vi "action controller.vi"(10 "Box Sensor":bool, 11 "Buttons":bool[](array[boolean])) -> ()   [LabVIEW 2018]
uses:
  First Power Up 2018 current/Robot Global Data.vi
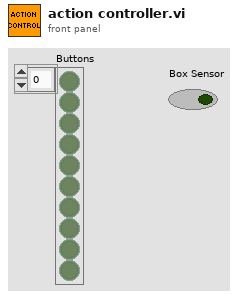
[diagram p1: front panel]
types:
  T1 = enum16{"Pickup", "Store", "Lift", "Straight Lift"}
  T2 = cluster{"Buttons[0]":bool, "Buttons[1]":bool, "Buttons[2]":bool, "Buttons[3]":bool, "Buttons[4]":bool, "Buttons[5]":bool, "Buttons[6]":bool, "Buttons[7]":bool, "Buttons[8]":bool}
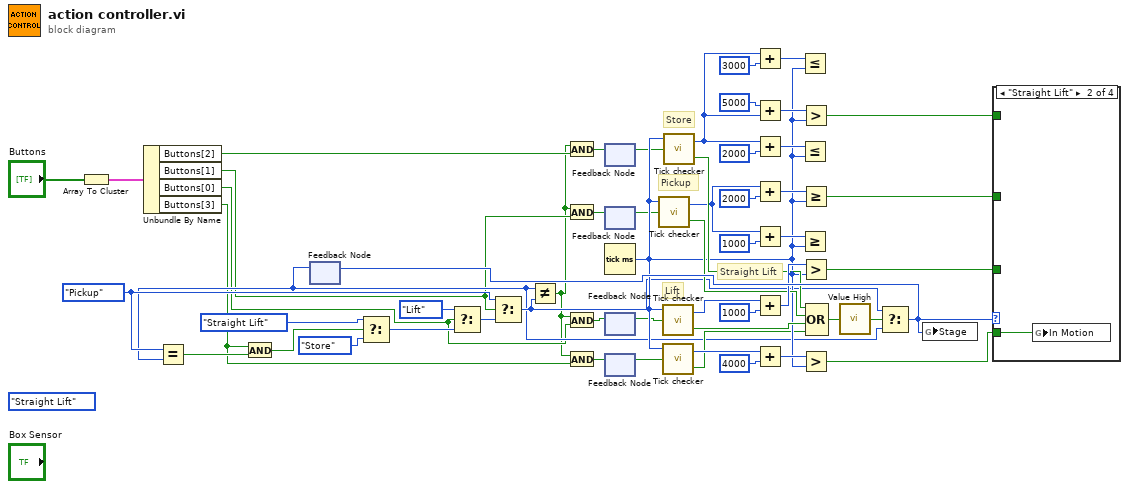
[diagram p0: block diagram]
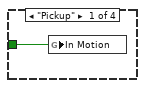
[diagram p2: hidden frame]
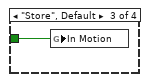
[diagram p3: hidden frame]
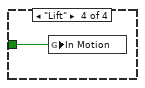
[diagram p4: hidden frame]
diagram:
  w44 = T1."Pickup" ("Stage")
  (unwired) T1."Straight Lift" ("Stage")
  # "Straight Lift"
  # "Lift"
  # "Pickup"
  # "Store"
  n1 = Array To Cluster(array="Buttons") -> (cluster=w54:T2)
  n2 = Unbundle By Name(w54) -> ("Buttons[2]"=w13:bool, "Buttons[1]"=w9:bool, "Buttons[0]"=w6:bool, "Buttons[3]"=w3:bool)
  n3 = feedback #1() -> (w14:T1)  [unwired: 1 in]
  n4 = Equal?(x=w44, y=w14) -> (x = y?=w46:bool)
  n5 = And(x=w3, y=w46) -> (x .and. y?=w45:bool)
  n6 = Select(t=T1."Straight Lift" ("Stage"), s=w45, f=T1."Store" ("Stage")) -> (s? t:f=w51:T1)
  n7 = Select(t=T1."Lift" ("Stage"), s=w6, f=w51) -> (s? t:f=w50:T1)
  n8 = Select(t=w44, s=w9, f=w50) -> (s? t:f=w15:T1)
  n9 = Not Equal?(x=w14, y=w15) -> (x != y?=w2:bool)
  n10 = And(x=w2, y=w13) -> (x .and. y?=w12:bool)
  n11 = And(x=w2, y=w9) -> (x .and. y?=w10:bool)
  n12 = And(x=w2, y=w6) -> (x .and. y?=w7:bool)
  n13 = And(x=w2, y=w3) -> (x .and. y?=w4:bool)
  n14 = feedback-in #2(w12) -> ()
  n15 = feedback #2() -> (w11:bool)  [unwired: 1 in]
  n16 = feedback #3() -> (w8:bool)  [unwired: 1 in]
  n17 = feedback-in #3(w10) -> ()
  n18 = Tick Count (ms)() -> (millisecond timer value=w18:u32)
  n19 = feedback #4() -> (w5:bool)  [unwired: 1 in]
  n20 = feedback-in #4(w7) -> ()
  n21 = feedback #5() -> (w1:bool)  [unwired: 1 in]
  n22 = feedback-in #5(w4) -> ()
  n23 = call "Tick checker.vi"("Start Sequence"=w8, "millisecond timer value"=w18) -> ("Out"=w21:bool, "Sequence time"=w22:u32)  [unwired: 1 in]
  n24 = call "Tick checker.vi"("Start Sequence"=w5, "millisecond timer value"=w18) -> ("Out"=w19:bool, "Sequence time"=w20:u32)  [unwired: 1 in]
  n25 = call "Tick checker.vi"("Start Sequence"=w1, "millisecond timer value"=w18) -> ("Out"=w16:bool, "Sequence time"=w17:u32)  [unwired: 1 in]
  n26 = call "Tick checker.vi"("Start Sequence"=w11, "millisecond timer value"=w18) -> ("Out"=w23:bool, "Sequence time"=w24:u32)  [unwired: 1 in]
  n27 = Add(x=w24, y=u32 3000) -> (x+y=w42:u32)
  n28 = Add(x=u32 5000 ("y"), y=w24) -> (x+y=w28:u32)
  n29 = Add(x=w24, y=u32 2000) -> (x+y=w53:u32)
  n30 = Add(x=w22, y=u32 2000) -> (x+y=w39:u32)
  n31 = Add(x=w22, y=u32 1000) -> (x+y=w40:u32)
  n32 = Add(x=w20, y=u32 1000) -> (x+y=w36:u32)
  n33 = Add(x=w17, y=u32 4000) -> (x+y=w33:u32)
  n34 = Less Or Equal?(x=w42, y=w18) -> ()  [unwired: 1 out]
  n35 = Less Or Equal?(x=w53, y=w18) -> ()  [unwired: 1 out]
  n36 = Greater Or Equal?(x=w40, y=w18) -> ()  [unwired: 1 out]
  n37 = Greater?(x=w28, y=w18) -> (0:w29:bool)
  n38 = Greater Or Equal?(x=w39, y=w18) -> (x >= y?=w31:bool)
  n39 = Greater?(x=w36, y=w18) -> (0:w32:bool)
  n40 = Greater?(x=w33, y=w18) -> (0:w30:bool)
  n41 = Compound Arithmetic op=OR(w23, w21, w19, w16) -> (w25:bool)
  n42 = call "Value High.vi"("In"=w25) -> ("Out"=w26:bool)
  n43 = Select(t=w15, s=w26, f=w14) -> (s? t:f=w37:T1)
  n44 = feedback-in #1(w37) -> ()
  n45 = global write "Robot Global Data.vi" "Stage"(w37) -> ()
  n46 = case shown="\"Straight Lift\"" w37 {
    tunnel: w32 -> [_ _ _ w59]
    tunnel: w31 -> [w56 _ _ _]
    tunnel: w30 -> [_ w57 _ _]
    tunnel: w29 -> [_ _ w58 _]
    frame "Pickup" {
      n47 = global write "Robot Global Data.vi" "In Motion"(w56) -> ()
    }
    frame "Straight Lift" {
      n48 = global write "Robot Global Data.vi" "In Motion"(w57) -> ()
    }
    frame "Store", Default {
      n49 = global write "Robot Global Data.vi" "In Motion"(w58) -> ()
    }
    frame "Lift" {
      n50 = global write "Robot Global Data.vi" "In Motion"(w59) -> ()
    }
  }
